vi "dummy_mod.vi"(4 "error in":errorcluster, 6 "Request data":variant, 7 "Request":string) -> (0 "error out":errorcluster, 2 "Response data":variant)   [LabVIEW 2018]
panel:
  out "Python session":refnum<k35>
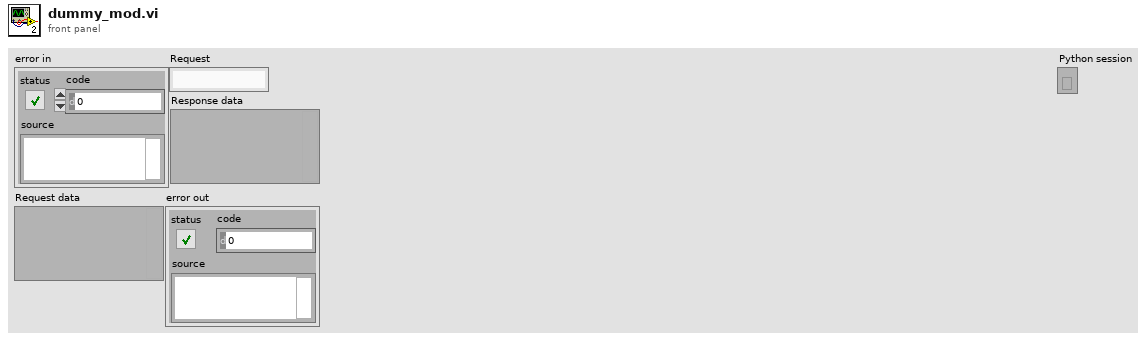
[diagram p1: front panel]
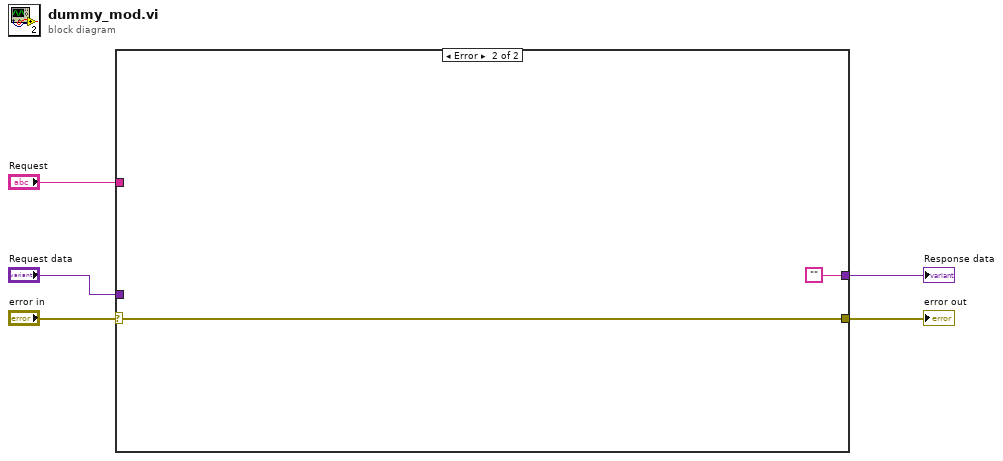
[diagram p0: block diagram]
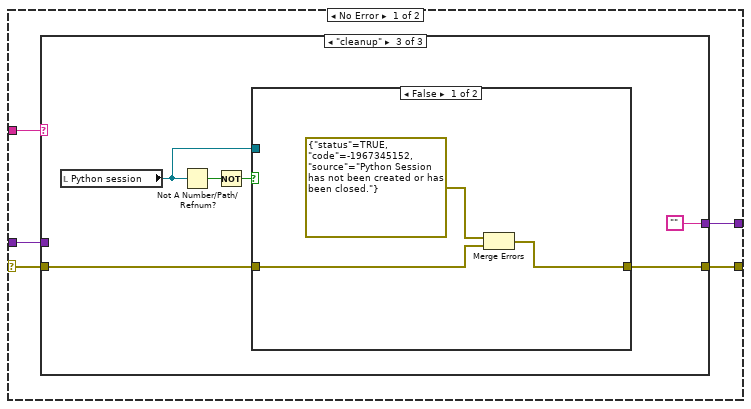
[diagram p2: hidden frame]
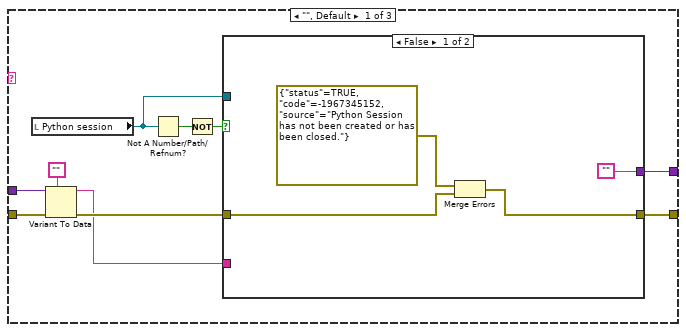
[diagram p3: hidden frame]
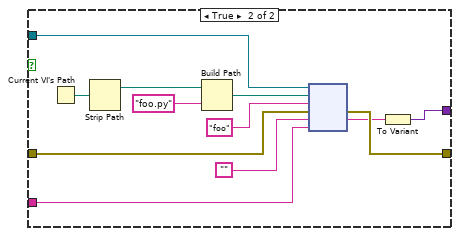
[diagram p4: hidden frame]
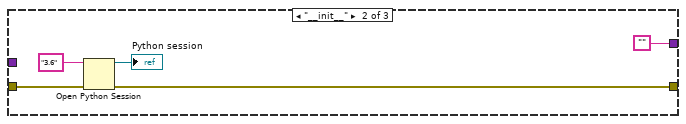
[diagram p5: hidden frame]
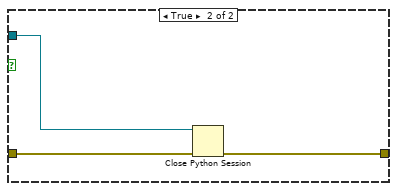
[diagram p6: hidden frame]
diagram:
  n1 = case shown="Error" "error in" {
    selector: "error in" -> [w9 w55]
    tunnel: [w7 w55] -> w4
    tunnel: "Request" -> [w10 _]
    tunnel: "Request data" -> [w8 _]
    tunnel: [w6 ""] -> w1
    frame No Error {
      n2 = case shown="\"cleanup\"" w10 {
        tunnel: w9 -> [w20 w41 w45]
        tunnel: w8 -> [w19 _ _]
        tunnel: [w14 w38 w44] -> w7
        tunnel: [w11 "" ""] -> w6
        frame "", Default {
          n3 = local read "Python session"() -> (w13:refnum<k35>)
          n4 = Variant To Data(error in=w20, type="", Variant=w19) -> (data=w12:string, error out=w15:errorcluster)
          n5 = Not A Number/Path/Refnum?(number/path/refnum=w13) -> (NaN/Path/Refnum?=w17:bool)
          n6 = Not(x=w17) -> (.not. x?=w16:bool)
          n7 = case shown="False" w16 {
            tunnel: w15 -> [w24 w30]
            tunnel: [w22 w27] -> w14
            tunnel: w13 -> [_ w36]
            tunnel: w12 -> [_ w28]
            tunnel: ["" w25] -> w11
            frame False {
              n8 = Merge Errors(errorcluster {"status"=TRUE, "code"=-1967345152, "source"="Python Session has not been created or has been closed."} ("error constant"), w24) -> (w22:errorcluster)
            }
            frame True {
              n9 = Current VI's Path() -> (path=w34:path)
              n10 = Strip Path(path=w34) -> (stripped path=w35:path)  [unwired: 1 out]
              n11 = Build Path(base path=w35, name or relative path="foo.py") -> (appended path=w32:path)
              n12 = node(w36, w32, "foo" ("function name"), w30, "", w28) -> (w27:errorcluster, w26:string)  [unwired: 1 in, 3 out]
              n13 = To Variant(anything=w26) -> (Variant=w25:variant)
            }
          }
        }
        frame "__init__" {
          n14 = Open Python Session(python version="3.6" ("Python version"), 3:w41) -> (session out=→"Python session":refnum<k35>, error out=w38:errorcluster)  [unwired: 1 in]
        }
        frame "cleanup" {
          n15 = local read "Python session"() -> (w47:refnum<k35>)
          n16 = Not A Number/Path/Refnum?(number/path/refnum=w47) -> (NaN/Path/Refnum?=w46:bool)
          n17 = Not(x=w46) -> (.not. x?=w43:bool)
          n18 = case shown="False" w43 {
            tunnel: w45 -> [w50 w53]
            tunnel: [w48 w51] -> w44
            tunnel: w47 -> [_ w52]
            frame False {
              n19 = Merge Errors(errorcluster {"status"=TRUE, "code"=-1967345152, "source"="Python Session has not been created or has been closed."} ("error constant"), w50) -> (w48:errorcluster)
            }
            frame True {
              n20 = Close Python Session(session in=w52, error in=w53) -> (11:w51:errorcluster)
            }
          }
        }
      }
    }
    frame Error {
    }
  }
  "Response data" <- w1
  "error out" <- w4
